vi "losslessCompression.vi"(5 "Image":T1, 7 "error in (no error)":errorcluster) -> (0 "Data String":string, 3 "error out":errorcluster)   [LabVIEW 2011]
uses:
  IMAQ Image.ctl
panel:
  out "length":i32
  out "number of replacements":i32
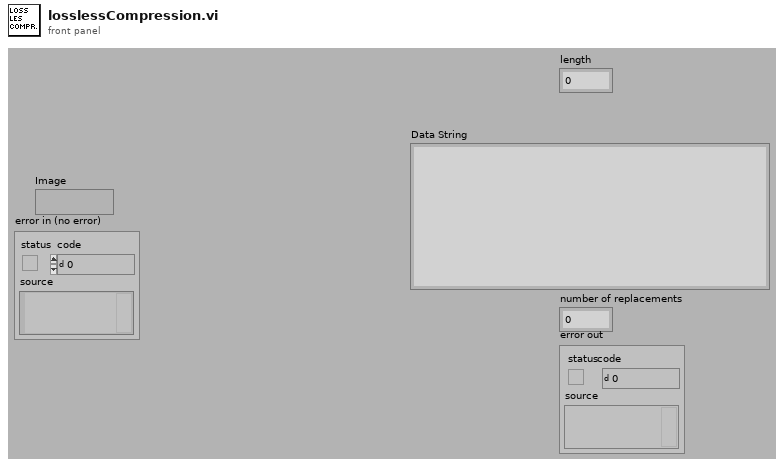
[diagram p1: front panel]
types:
  T1 = typedef "IMAQ Image.ctl" = refnum<image>
  T2 = typedef "Image Type" = u32
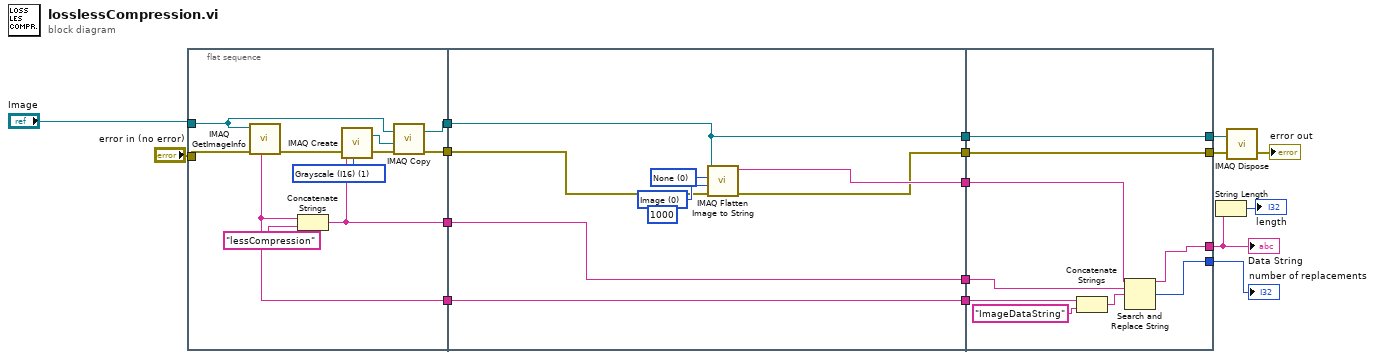
[diagram p0: block diagram]
diagram:
  n1 = flat-sequence {
    tunnel: "error in (no error)" -> [w24]
    tunnel: "Image" -> [w26]
    tunnel: [w25] -> w10
    tunnel: [w21] -> w6
    tunnel: [w20] -> w4
    tunnel: [w19] -> w3
    tunnel: w10 -> [w34]
    tunnel: [w31] -> w9
    tunnel: [w34] -> w8
    tunnel: [w33] -> w7
    tunnel: w6 -> [w32]
    tunnel: [w30] -> w5
    tunnel: w4 -> [w30]
    tunnel: w3 -> [w29]
    tunnel: [w29] -> w2
    tunnel: [w44] -> w12
    tunnel: [w45] -> w14
    tunnel: [w40] -> w17
    tunnel: [w39] -> w1
    tunnel: w9 -> [w45]
    tunnel: w8 -> [w44]
    tunnel: w7 -> [w38]
    tunnel: w5 -> [w42]
    tunnel: w2 -> [w41]
    frame #0 {
      w28 = T2 1 items=["Grayscale (U8)", "Grayscale (I16)", "Grayscale (SGL)", "Complex (CSG)", "RGB (U32)", "HSL (U32)", "RGB (U64)", "Grayscale (U16)"] ("Image Type")
      n2 = call "IMAQ GetImageInfo"("error in (no error)"=w24, "Image"=w26) -> ("error out"=w23:errorcluster, "Image Name"=w19:string)  [unwired: 2 in, 6 out]
      n3 = Concatenate Strings(w19, "lessCompression" ("string")) -> (w20:string)
      n4 = call "IMAQ Create"("Image Name"=w20, "Image Type"=w28, "error in (no error)"=w23) -> ("New Image"=w27:T1, "error out"=w22:errorcluster)  [unwired: 2 in]
      n5 = call "IMAQ Copy"("error in (no error)"=w22, "Image Dst"=w27, "Image Src"=w26) -> ("error out"=w21:errorcluster, "Image Dst Out"=w25:T1)  [unwired: 3 in]
    }
    frame #1 {
      w35 = 0 items=["Image", "Image and Vision Info", "Reference to Image"] ("Type of Flatten (Image and Vision Info)")
      (unwired) 1000 ("Quality (750)")
      w36 = 0 items=["None", "JPEG", "PACKED BINARY"] ("Compression (None)")
      n6 = call "IMAQ Flatten Image to String"("error in (no error)"=w32, "Type of Flatten (Image and Vision Info)"=w35, "Compression (None)"=w36, "Image"=w34) -> ("error out"=w31:errorcluster, "Data String"=w33:string)  [unwired: 6 in]
    }
    frame #2 {
      n7 = Concatenate Strings(w41, "ImageDataString" ("replace string (\"\")")) -> (w43:string)
      n8 = Search and Replace String(input string=w38, search string=w42, replace string=w43) -> (result string=w39:string, number of replacements=w40:i32)  [unwired: 5 in, 2 out]
    }
  }
  n9 = String Length(string=w1) -> (length=→"length":i32)
  n10 = call "IMAQ Dispose"("Image"=w12, "error in (no error)"=w14) -> ("error out"=→"error out":errorcluster)  [unwired: 4 in]
  "Data String" <- w1
  "number of replacements" <- w17
